vi "ex1a.vi"() -> ()   [LabVIEW 2022 SP3]
panel:
  out "Array":i32[][](array[numeric])
  in  "dimension size":i32
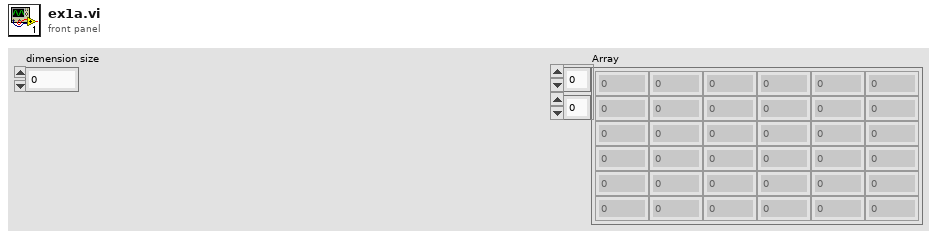
[diagram p1: front panel]
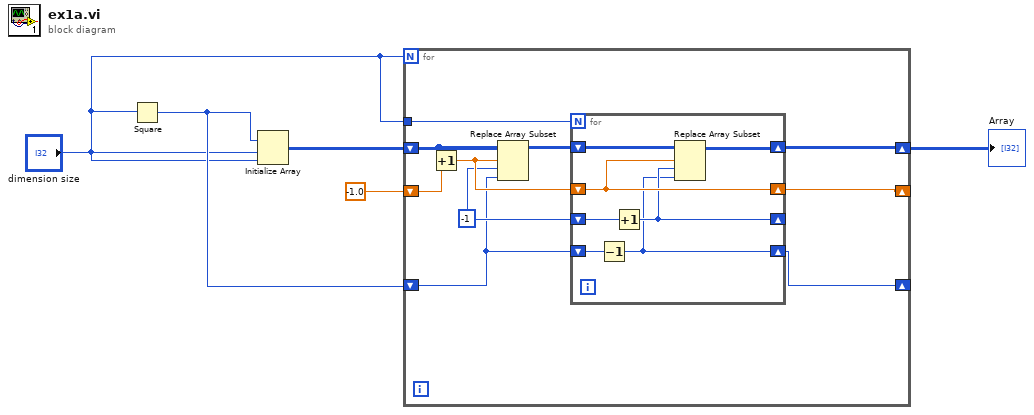
[diagram p0: block diagram]
diagram:
  n1 = Square(x="dimension size") -> (x^2=w4:i32)
  n2 = Initialize Array(w4, "dimension size", "dimension size") -> (w5:i32[][])
  n3 = for {
    N: "dimension size" -> [_]
    shift-right: [w10] -> w2
    shift-left: w5 -> [w11]
    shift-right: [w6] -> _
    shift-left: w4 -> [w7]
    shift-right: [w9] -> _
    shift-left: -1.0 -> [w14]
    tunnel: "dimension size" -> [w8]
    w12 = -1
    n4 = Increment(x=w14) -> (x+1=w13:dbl)
    n5 = Replace Array Subset(array=w11, new element=w7, index (row)=w13, index (col)=w12) -> ()  [unwired: 1 out]
    n6 = for {
      N: w8 -> [_]
      shift-right: [w17] -> w9
      shift-left: w13 -> [w17]
      shift-right: [w16] -> _
      shift-left: w12 -> [w21]
      shift-right: [w18] -> w10
      shift-left: w11 -> [w20]
      shift-right: [w15] -> w6
      shift-left: w7 -> [w19]
      n7 = Decrement(x=w19) -> (x-1=w15:i32)
      n8 = Increment(x=w21) -> (x+1=w16:i32)
      n9 = Replace Array Subset(array=w20, new element=w15, index (row)=w17, index (col)=w16) -> (w18:i32[][])
    }
  }
  "Array" <- w2
